vi "DrawCrossHairs.vi"(11 "Image In":T1) -> (3 "Image Out":T1)   [LabVIEW 2012]
uses:
  <vilib>/vision/Image Controls.llb/IMAQ Image.ctl
  <vilib>/vision/NI_Vision_Development_Module.lvlib
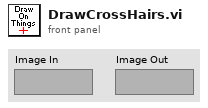
[diagram p1: front panel]
types:
  T1 = typedef "IMAQ Image.ctl" = refnum<image>
  T2 = cluster{"Red or Hue value":u8, "Green or Sat value":u8, "Blue or Luma or Val or Inten value":u8}
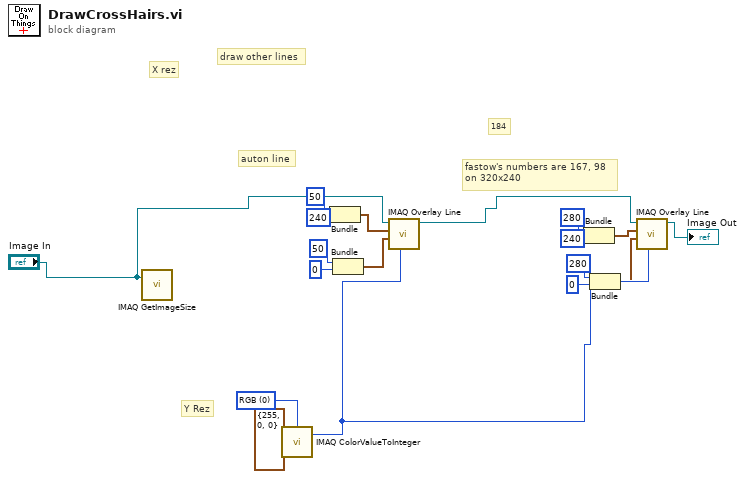
[diagram p0: block diagram]
diagram:
  w18 = u16 0 items=["RGB", "HSL", "HSV", "HSI"] ("Color Mode")
  # "auton line"
  # "fastow's numbers are 167, 98\non 320x240"
  # "184"
  # "draw other lines"
  # "Y Rez"
  # "X rez"
  n1 = call "IMAQ GetImageSize"("Image"="Image In") -> ()  [unwired: 3 in, 3 out]
  n2 = call "IMAQ ColorValueToInteger"("Color Value"=T2 {"Red or Hue value"=255, "Green or Sat value"=0, "Blue or Luma or Val or Inten value"=0}, "Color Mode"=w18) -> ("U32 value"=w14:u32)  [unwired: 3 in, 3 out]
  n3 = Bundle(50, 240) -> (w1:cluster{i32, i32})  [unwired: 1 in]
  n4 = Bundle(50, 0) -> (w2:cluster{i32, i32})  [unwired: 1 in]
  n5 = call "IMAQ Overlay Line"("Color"=w14, "End Point"=w2, "Start Point"=w1, "Image"="Image In") -> ("Image Out"=w13:T1)  [unwired: 6 in, 1 out]
  n6 = Bundle(280, 240) -> (w3:cluster{i32, i32})  [unwired: 1 in]
  n7 = Bundle(280, 0) -> (w4:cluster{i32, i32})  [unwired: 1 in]
  n8 = call "IMAQ Overlay Line"("Color"=w14, "End Point"=w4, "Start Point"=w3, "Image"=w13) -> ("Image Out"=→"Image Out":T1)  [unwired: 6 in, 1 out]
